vi "CalculateCaseStructureBoundingBox.vi"(8 "Error In":errorcluster, 10 "Items to enclose in case structure":refnum<vi>[](array[refnum]), 11 "VI reference":refnum<vi>) -> (0 "Error Out":errorcluster, 2 "Current bounding box position":cluster{"Left":i32, "Top":i32}, 3 "Size of bounding box for items":T1)   [LabVIEW 2017, in "ErrorStructureDrawer.lvlib"]
doc: "Calculate the height and width of a bounding box for items that will go inside the case structure, plus any extra vertical height needed to also contain controls and indicators."
uses:
  ErrorStructureDrawer.lvlib
  <vilib>/Utility/miscctls.llb/LVBoundsTypeDef.ctl
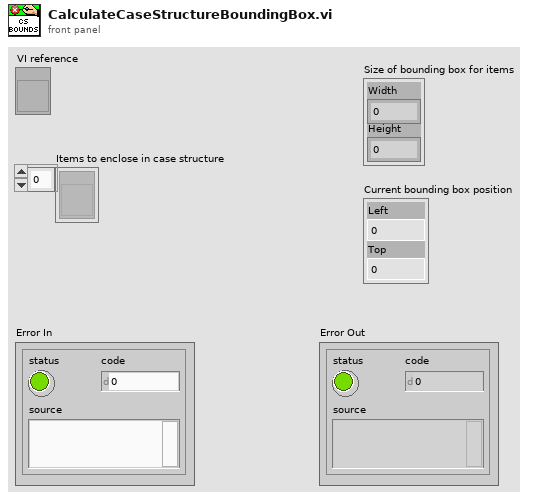
[diagram p1: front panel]
types:
  T1 = typedef "LVBoundsTypeDef.ctl" = cluster{"Width":u32, "Height":u32}
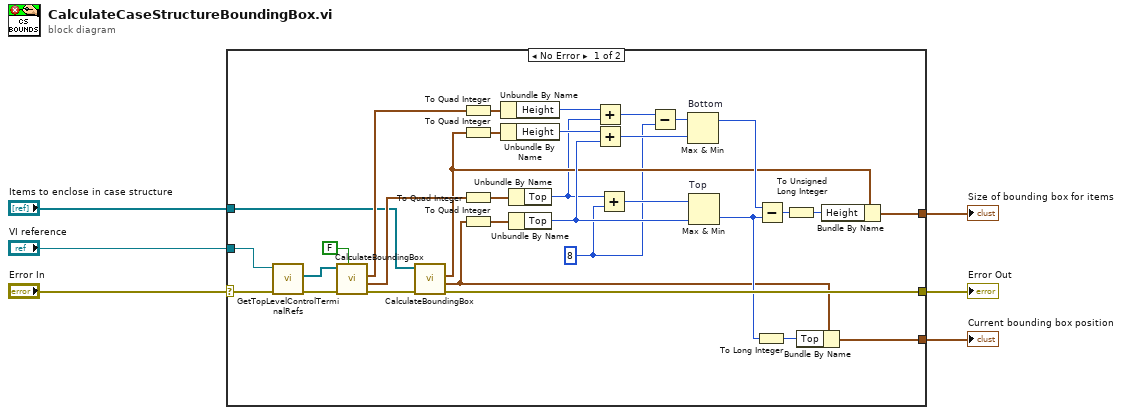
[diagram p0: block diagram]
diagram:
  n1 = case shown="No Error" "Error In" {
    selector: "Error In" -> [w19 w39]
    tunnel: [w7 _] -> w6
    tunnel: [w38 _] -> w5
    tunnel: "VI reference" -> [w29 _]
    tunnel: "Items to enclose in case structure" -> [w17 _]
    tunnel: [w18 w39] -> w1
    frame No Error {
      w9 = i64 8 ("y")
      n2 = call "GetTopLevelControlTerminalRefs.vi"("error in (no error)"=w19, "VI ref in"=w29) -> ("error out"=w37:errorcluster, "Control terminals on top-level"=w16:refnum<vi>[])  [unwired: 7 in, 1 out]
      n3 = call "CalculateBoundingBox.vi"("Include labels etc? [t]"=FALSE, "error in (no error)"=w37, "Items"=w16) -> ("error out"=w36:errorcluster, "Current bounding box position"=w25:cluster{"Left":i32, "Top":i32}, "Size of bounding box for items"=w28:T1)  [unwired: 5 in, 1 out]
      n4 = call "CalculateBoundingBox.vi"("error in (no error)"=w36, "Items"=w17) -> ("error out"=w18:errorcluster, "Current bounding box position"=w8:cluster{"Left":i32, "Top":i32}, "Size of bounding box for items"=w20:T1)  [unwired: 6 in, 1 out]
      n5 = To Quad Integer(1:w28) -> (0:w27:cluster{"Width":i64, "Height":i64})
      n6 = To Quad Integer(1:w20) -> (0:w26:cluster{"Width":i64, "Height":i64})
      n7 = To Quad Integer(1:w25) -> (0:w24:cluster{"Left":i64, "Top":i64})
      n8 = To Quad Integer(1:w8) -> (0:w23:cluster{"Left":i64, "Top":i64})
      n9 = Unbundle By Name(w27) -> ("Height"=w30:i64)
      n10 = Unbundle By Name(w26) -> ("Height"=w31:i64)
      n11 = Unbundle By Name(w24) -> ("Top"=w14:i64)
      n12 = Unbundle By Name(w23) -> ("Top"=w32:i64)
      n13 = Add(x=w30, y=w14) -> (x+y=w12:i64)
      n14 = Add(x=w31, y=w32) -> (x+y=w33:i64)
      n15 = Add(x=w14, y=w9) -> (x+y=w13:i64)
      n16 = Subtract(x=w12, y=w9) -> (x-y=w11:i64)
      n17 = Max & Min "Bottom"(x=w11, y=w33) -> (max(x,y)=w34:i64)  [unwired: 1 out]
      n18 = Max & Min "Top"(x=w13, y=w32) -> (min(x,y)=w15:i64)  [unwired: 1 out]
      n19 = To Long Integer(number=w15) -> (32bit integer=w22:i32)
      n20 = Subtract(x=w34, y=w15) -> (x-y=w35:i64)
      n21 = To Unsigned Long Integer(number=w35) -> (unsigned 32bit integer=w21:u32)
      n22 = Bundle By Name(cluster=w8, "Top"=w22) -> (w7:cluster{"Left":i32, "Top":i32})
      n23 = Bundle By Name(cluster=w20, "Height"=w21) -> (w38:T1)
    }
    frame Error {
    }
  }
  "Current bounding box position" <- w6
  "Size of bounding box for items" <- w5
  "Error Out" <- w1
